vi "Find Project Dependencies.vi"(0 "Project Path in":path, 1 "Load Stored Targets?(T)":bool=TRUE, 2 "Exclude Own Project Files?(T)":bool=TRUE, 5 "Dependency Source Plugins":refnum<class "Dependency Source.lvclass">[](array[class]), 11 "Error In":errorcluster, 12 "To Lower Case?(T)":bool=TRUE) -> (3 "Plugin Load Success? Array":bool[](array[boolean]), 4 "Project Path dub":path, 6 "Found Internal Dependencies":T1[](array[typedef]), 8 "Found External Dependencies":T1[](array[typedef]), 10 "Unhandled Targets":T1[](array[typedef]), 15 "Error Out":errorcluster)   [LabVIEW 2019, in "Project.Dependencies Finder.lvlib"]
doc: "Parse a project file for internal and external dependencies.\n\nInternal dependencies are expected to have 'paths' like vi.lib\\ and should be found inside the LabVIEW folder.\nExternal dependencies are identified by unique folder names.\n\n2020-11-13: Henrik Dueholm Hansen"
uses:
  Project.Dependencies Finder.lvlib
  Ctl/Ctl_Dependency Element.ctl
  Dependency Source/Dependency Source.lvclass
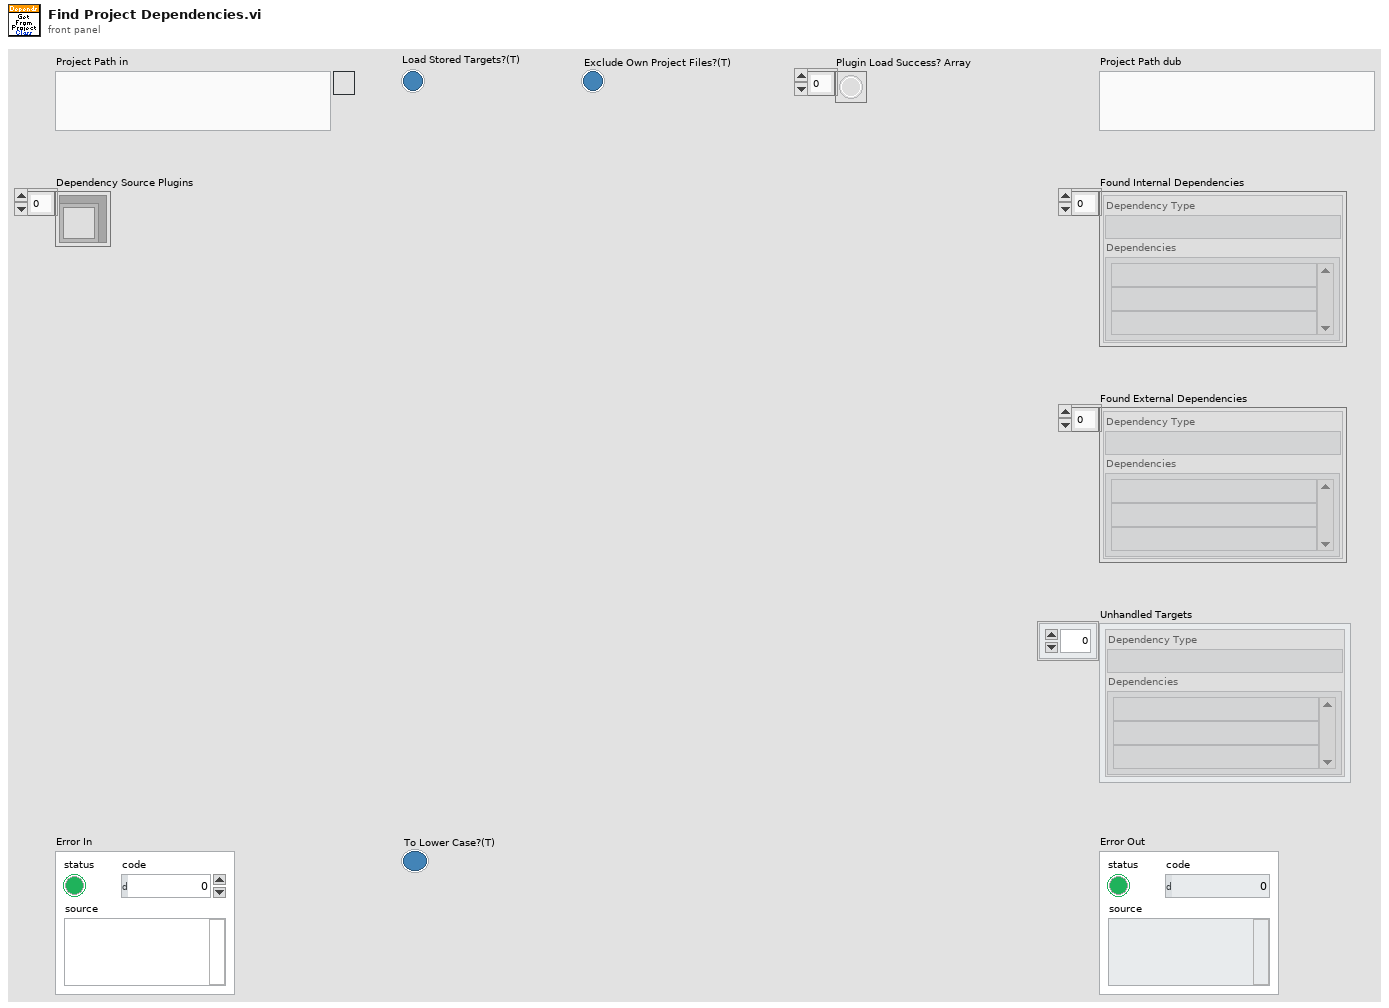
[diagram p1: front panel]
types:
  T1 = typedef "Project.Dependencies Finder.lvlib/Ctl_Dependency Element.ctl" = cluster{"Dependency Type":string, "Dependencies":string[]}
  T2 = typedef "Project.Dependencies Finder.lvlib/Ctl_External Target Element.ctl" = cluster{"Target Source":string, "External Target Map":map{string, string}}
  T3 = typedef "Project.Dependencies Finder.lvlib/Ctl_Internal Target Element.ctl" = cluster{"Target Source":string, "Internal Target Map":map{string, string}}
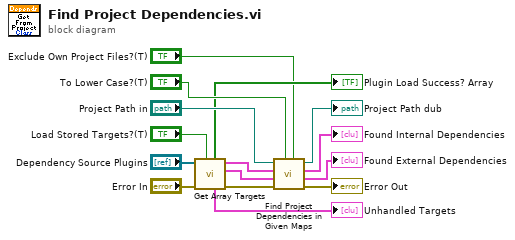
[diagram p0: block diagram]
diagram:
  n1 = call "Get Array Targets.vi"("Load Stored Targets?(T)"="Load Stored Targets?(T)", "error in (no error)"="Error In", "Dependency Sources"="Dependency Source Plugins") -> ("error out"=w10:errorcluster, "External Targets"=w11:T2[], "Internal Targets"=w12:T3[], "Unhandled Targets"=→"Unhandled Targets":T1[], "Success? Array"=→"Plugin Load Success? Array":bool[])  [unwired: 3 in, 1 out]
  n2 = call "Find Project Dependencies in Given Maps.vi"("Exclude Own Project Files?(T)"="Exclude Own Project Files?(T)", "To Lower Case?(T)"="To Lower Case?(T)", "Error In"=w10, "External Targets"=w11, "Internal Targets"=w12, "Project Path in"="Project Path in") -> ("Error Out"=→"Error Out":errorcluster, "Found External Dependencies"=→"Found External Dependencies":T1[], "Found Internal Dependencies"=→"Found Internal Dependencies":T1[], "Project Path dub"=→"Project Path dub":path)  [unwired: 2 in]
